vi "MEASUAMENT.vi"(8 "error in (no error)":errorcluster, 9 "Manual Range (1.00)":dbl=1.0 format="%_3f", 10 "Function (0: DC Voltage)":u16(ring) items=["DC Voltage", "AC Voltage", "2 - Wire Resistance", "2 -Wire Resistance low power", "4 - Wire Resistance", "4- Wire Resistance low power", "DC Current", "AC Current", "CLAMP DC", "CLAMP AC", "Frequency", "Continuity", "Diode Checking"], 11 "VISA resource name":refnum<visa-resource-name>) -> (0 "error out":errorcluster, 2 "Measurement":dbl, 3 "VISA resource name out":refnum<visa-resource-name>)   [LabVIEW 2017]
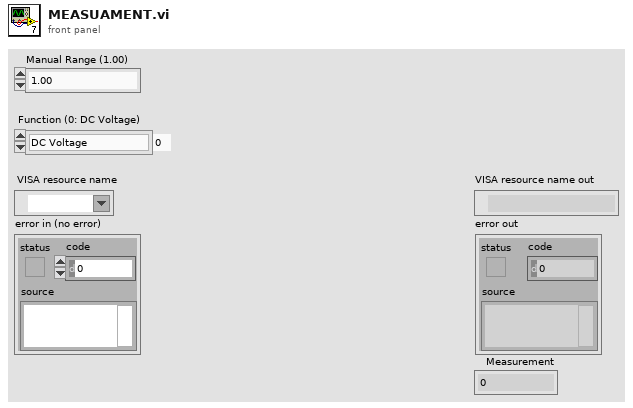
[diagram p1: front panel]
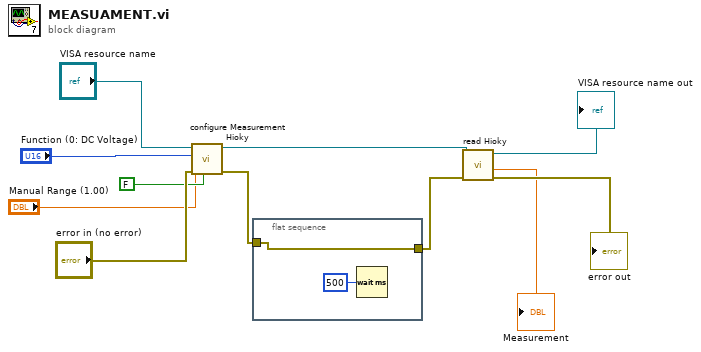
[diagram p0: block diagram]
diagram:
  n1 = call "configure Measurement Hioky.vi"("Enable Auto Range (T: Enable)"=FALSE, "error in (no error)"="error in (no error)", "Manual Range (1.00)"="Manual Range (1.00)", "Function (0: DC Voltage)"="Function (0: DC Voltage)", "VISA resource name"="VISA resource name") -> ("error out"=w5:errorcluster, "VISA resource name out"=w11:refnum<visa-resource-name>)  [unwired: 5 in]
  n2 = flat-sequence {
    tunnel: w5 -> [w13]
    tunnel: [w13] -> w4
    frame #0 {
      n3 = Wait (ms)(milliseconds to wait=u32 500) -> ()  [unwired: 1 out]
    }
  }
  n4 = call "read Hioky.vi"("error in (no error)"=w4, "VISA resource name"=w11) -> ("error out"=→"error out":errorcluster, "Measurement"=→"Measurement":dbl, "VISA resource name out"=→"VISA resource name out":refnum<visa-resource-name>)  [unwired: 7 in]
